vi "LC-MISDK_Meas_Lvxy_LOEM.vi"(0 ".NET reference":refnum<k24>, 5 "comPort":i32, 11 "error in":errorcluster) -> (4 ".NET reference out":refnum<k24>, 6 "Lv":dbl, 8 "x":dbl, 10 "y":dbl, 13 "ReadLatestData Error":dbl format="%#_6f", 15 "error out":errorcluster)   [LabVIEW 2019]
uses:
  C:/Program Files (x86)/National Instruments/LabVIEW 2019/LC-MISDK.dll
  Program Files (x86)/National Instruments/LabVIEW 2019/LC-MISDK.dll
panel:
  out "Lv 2":dbl
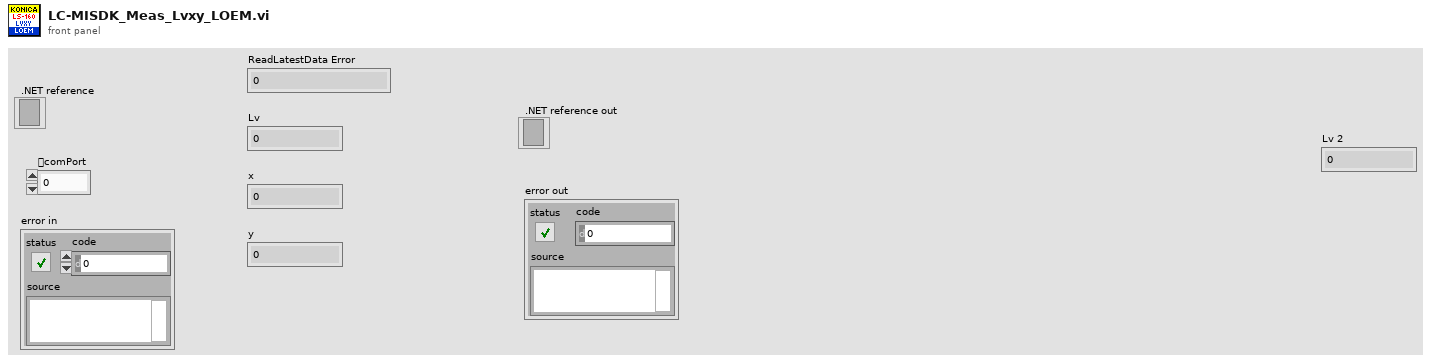
[diagram p1: front panel]
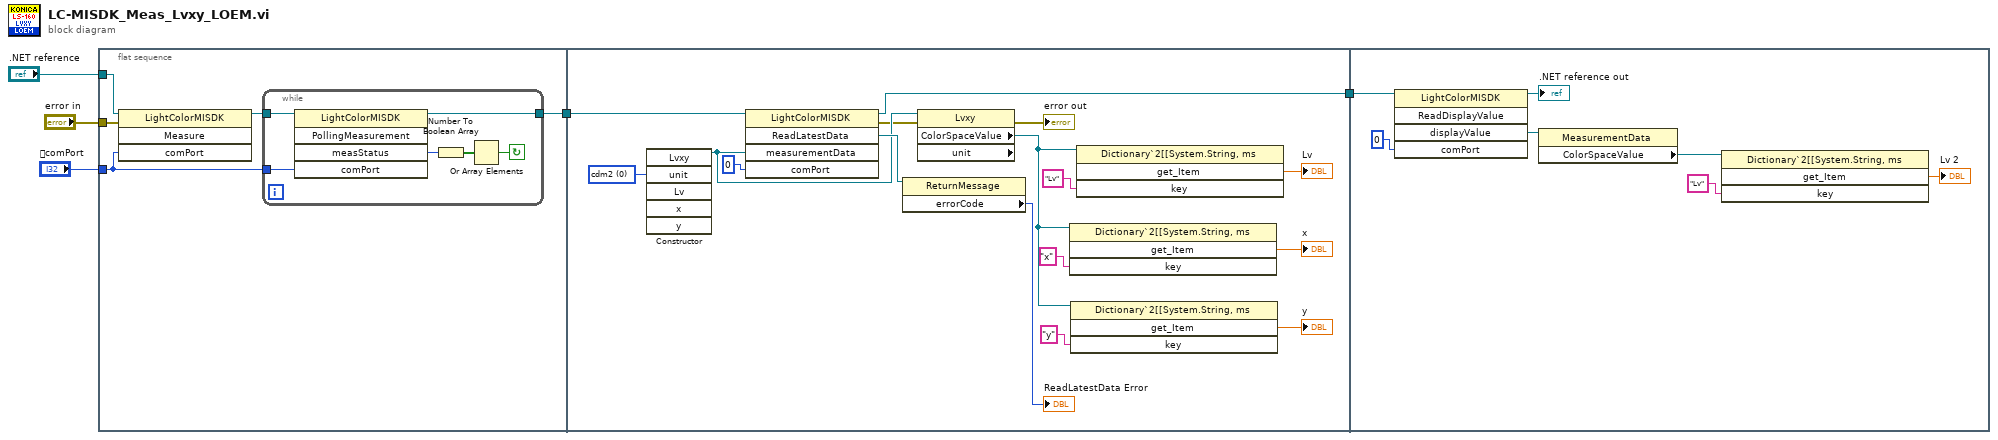
[diagram p0: block diagram]
diagram:
  n1 = flat-sequence {
    tunnel: ".NET reference" -> [w9]
    tunnel: "comPort" -> [w7]
    tunnel: [w10] -> w5
    tunnel: "error in" -> [w6]
    tunnel: w5 -> [w24]
    tunnel: [w22] -> w1
    tunnel: w1 -> [w39]
    frame #0 {
      n2 = invoke on="インボークノード" class="LightColorMISDK" method="Measure"(reference=w9, error in=w6, "comPort"=w7) -> (reference out=w8:refnum<k24>)  [unwired: 1 in, 3 out]
      n3 = while {
        tunnel: [w15] -> w10
        tunnel: w8 -> [w14]
        tunnel: w7 -> [w13]
        stop <- w11 continue-if-true
        n4 = invoke on="インボークノード" class="LightColorMISDK" method="PollingMeasurement"(reference=w14, "comPort"=w13) -> (reference out=w15:refnum<k24>, "measStatus"=w16:i32)  [unwired: 3 in, 3 out]
        n5 = Number To Boolean Array(number=w16) -> (Boolean array=w12:bool[])
        n6 = Or Array Elements(Boolean array=w12) -> (logical OR=w11:bool)
      }
    }
    frame #1 {
      w21 = 0 items=["cdm2", "other"] ("unit")
      n7 = constructor class="Lvxy"("unit"=w21) -> (reference out=w20:refnum<k24>)  [unwired: 6 in, 6 out]
      n8 = invoke on="インボークノード" class="LightColorMISDK" method="ReadLatestData"(reference=w24, "measurementData"=w20, "comPort"=0) -> (reference out=w22:refnum<k24>, error out=w19:errorcluster, "ReadLatestData"=w32:refnum<k24>)  [unwired: 2 in, 2 out]
      n9 = property on="プロパティノード" class="ReturnMessage"(reference=w32) -> ("errorCode"=→"ReadLatestData Error":i32)  [unwired: 1 in, 2 out]
      n10 = property class="Lvxy" props=["ColorSpaceValue", "unit"](reference=w20, error in=w19) -> (error out=→"error out":errorcluster, "ColorSpaceValue"=w17:refnum<k24>)  [unwired: 2 out]
      n11 = invoke class="Dictionary`2[[System.String, ms" method="get_Item"(reference=w17, "key"="x") -> ("get_Item"=→"x":dbl)  [unwired: 2 in, 3 out]
      n12 = invoke class="Dictionary`2[[System.String, ms" method="get_Item"(reference=w17, "key"="y") -> ("get_Item"=→"y":dbl)  [unwired: 2 in, 3 out]
      n13 = invoke class="Dictionary`2[[System.String, ms" method="get_Item"(reference=w17, "key"="Lv") -> ("get_Item"=→"Lv":dbl)  [unwired: 2 in, 3 out]
    }
    frame #2 {
      n14 = invoke class="LightColorMISDK" method="ReadDisplayValue"(reference=w39, "comPort"=0) -> (reference out=→".NET reference out":refnum<k24>, "displayValue"=w37:refnum<k24>)  [unwired: 3 in, 3 out]
      n15 = property class="MeasurementData"(reference=w37) -> ("ColorSpaceValue"=w34:refnum<k24>)  [unwired: 1 in, 2 out]
      n16 = invoke class="Dictionary`2[[System.String, ms" method="get_Item"(reference=w34, "key"="Lv") -> ("get_Item"=→"Lv 2":dbl)  [unwired: 2 in, 3 out]
    }
  }
